vi "Scriptee.vi"   [LabVIEW 2019]
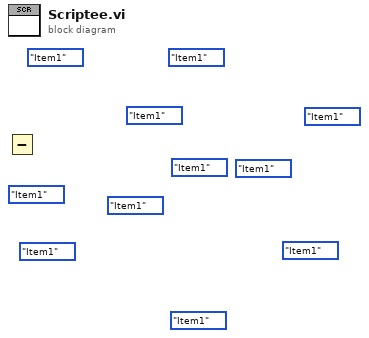
[diagram p0: block diagram]
diagram:
  (unwired) enum16{"Item1", "Item 2", "Item 3"}."Item1"
  (unwired) enum16{"Item1", "Item 2", "Item 3"}."Item1"
  (unwired) enum16{"Item1", "Item 2", "Item 3"}."Item1"
  (unwired) enum16{"Item1", "Item 2", "Item 3"}."Item1"
  (unwired) enum16{"Item1", "Item 2", "Item 3"}."Item1"
  (unwired) enum16{"Item1", "Item 2", "Item 3"}."Item1"
  (unwired) enum16{"Item1", "Item 2", "Item 3"}."Item1"
  (unwired) enum16{"Item1", "Item 2", "Item 3"}."Item1"
  (unwired) enum16{"Item1", "Item 2", "Item 3"}."Item1"
  (unwired) enum16{"Item1", "Item 2", "Item 3"}."Item1"
  (unwired) enum16{"Item1", "Item 2", "Item 3"}."Item1"
  n1 = Subtract() -> ()  [unwired: 2 in, 1 out]
  n2 = Subtract() -> ()  [unwired: 2 in, 1 out]
  n3 = Subtract() -> ()  [unwired: 2 in, 1 out]
  n4 = Subtract() -> ()  [unwired: 2 in, 1 out]
  n5 = Subtract() -> ()  [unwired: 2 in, 1 out]
  n6 = Subtract() -> ()  [unwired: 2 in, 1 out]
  n7 = Subtract() -> ()  [unwired: 2 in, 1 out]
  n8 = Subtract() -> ()  [unwired: 2 in, 1 out]
  n9 = Subtract() -> ()  [unwired: 2 in, 1 out]
  n10 = Subtract() -> ()  [unwired: 2 in, 1 out]
  n11 = Subtract() -> ()  [unwired: 2 in, 1 out]
